vi "sum_col.vi"(11 "Array":dbl[][](array[numeric])) -> (3 "row_vec(sum)":dbl[](array[numeric]))   [LabVIEW 2014]
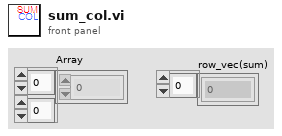
[diagram p1: front panel]
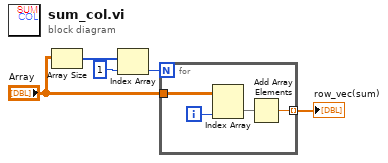
[diagram p0: block diagram]
diagram:
  n1 = Array Size(array="Array") -> (size(s)=w3:i32[])
  n2 = Index Array(array=w3, index=1) -> (element=w5:i32)
  n3 = for {
    N: w5 -> [_]
    tunnel: "Array" -> [w9]
    tunnel: [w7] -> w2 mode=indexing
    i -> [w6]
    n4 = Index Array(array=w9, index (col)=w6) -> (element=w8:dbl[])  [unwired: 1 in]
    n5 = Add Array Elements(numeric array=w8) -> (sum=w7:dbl)
  }
  "row_vec(sum)" <- w2
